vi "get_duration.vi"(8 "error in (no error)":errorcluster, 11 "ScanModeMG090624Camera in":refnum<class "ImagingModeMG090624Camera.lvclass">) -> (0 "error out":errorcluster, 2 "duration":dbl[unit], 3 "ScanModeMG090624Camera out":refnum<class "ImagingModeMG090624Camera.lvclass">)   [LabVIEW 2010, in "ImagingModeMG090624Camera.lvclass"]
uses:
  ImagingModeMG090624Camera.lvclass
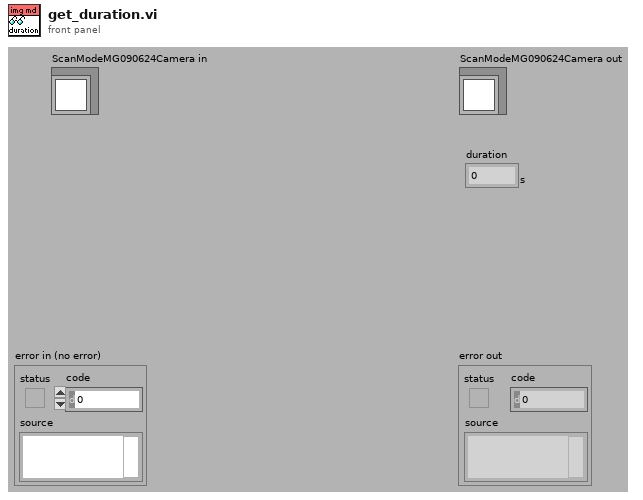
[diagram p1: front panel]
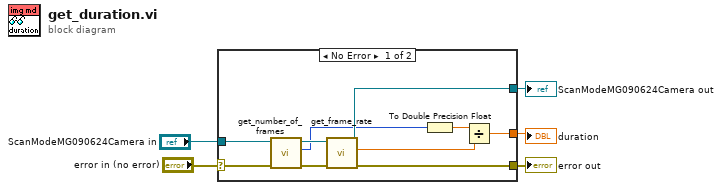
[diagram p0: block diagram]
diagram:
  n1 = case shown="No Error" "error in (no error)" {
    selector: "error in (no error)" -> [w9 w17]
    tunnel: [w8 w17] -> w4
    tunnel: [w11 w16] -> w2
    tunnel: "ScanModeMG090624Camera in" -> [w12 w16]
    tunnel: [w14 _] -> w3
    frame No Error {
      n2 = call-dynamic "get_number_of_frames.vi"("error in (no error)"=w9, "ScanModeMG090624Camera in"=w12) -> ("error out"=w10:errorcluster, "number of frames"=w7:i32, "ScanModeMG090624Camera out"=w13:refnum<class "ImagingModeMG090624Camera.lvclass">)  [unwired: 7 in]
      n3 = call-dynamic "get_frame_rate.vi"("error in (no error)"=w10, "ScanModeMG090624Camera in"=w13) -> ("error out"=w8:errorcluster, "frame rate"=w6:dbl[unit], "ScanModeMG090624Camera out"=w11:refnum<class "ImagingModeMG090624Camera.lvclass">)  [unwired: 7 in]
      n4 = To Double Precision Float(number=w7) -> (double precision float=w15:dbl)
      n5 = Divide(x=w15, y=w6) -> (x/y=w14:dbl[unit])
    }
    frame Error {
    }
  }
  "error out" <- w4
  "duration" <- w3
  "ScanModeMG090624Camera out" <- w2
